vi "TEST_L1_INITIALISATION_CHECK.vi"(5 "Serial Number":string="testFile", 6 "error in":errorcluster, 9 "VISA IN":T1={"AWG VISA"="AgilentGenerator1", "Oscilloscope  VISA "="AgilentOsciloscope", "Integration Board IP"="172.16.17.48", "connection ID"=refnum, "report out"=refnum, "report file path"=path "C:/Users/omartinez/Desktop/L0nL1_Results"}) -> (0 "error out":errorcluster, 3 "VISA OUT":T1={"AWG VISA"="AgilentGenerator1", "Oscilloscope  VISA "="AgilentOsciloscope", "Integration Board IP"="172.16.17.48", "connection ID"=refnum, "report out"=refnum, "report file path"=path "C:/Users/omartinez/Desktop/L0nL1_Results"})   [LabVIEW 2012]
uses:
  <vilib>/Utility/NIReport.llb/NI_report.lvclass
  <vilib>/Utility/NIReport.llb/HTML/NI_HTML.lvclass
panel:
  in  "Default register":u16[](array[numeric])=[6826, 18761, 18761, 18761, 30576, 383, 13312]
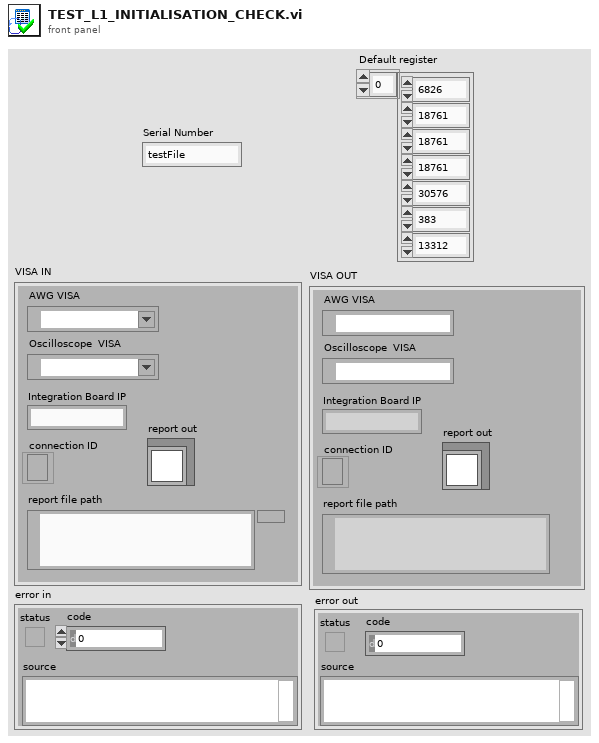
[diagram p1: front panel]
types:
  T1 = cluster{"AWG VISA":refnum<visa-resource-name>, "Oscilloscope  VISA ":refnum<visa-resource-name>, "Integration Board IP":string, "connection ID":refnum<k5>, "report out":refnum<class "NI_report.lvclass">, "report file path":path}
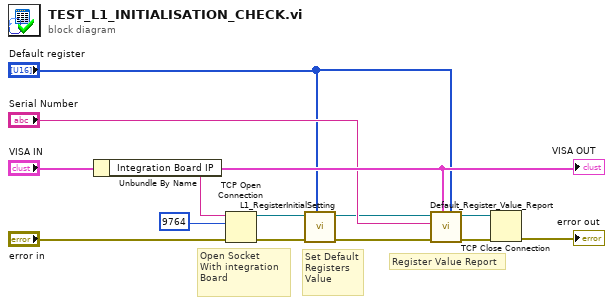
[diagram p0: block diagram]
diagram:
  # "Set Default\nRegisters\nValue"
  # "Open Socket\nWith integration \nBoard"
  # "Register Value Report"
  n1 = Unbundle By Name("VISA IN") -> ("Integration Board IP"=w8:string)
  n2 = TCP Open Connection(address=w8, remote port or service name=9764, error in (no error)="error in") -> (connection ID=w3:refnum<k5>, error out=w5:errorcluster)  [unwired: 2 in]
  n3 = call "L1_RegisterInitialSetting.vi"("REG ARRAy"="Default register", "error in"=w5, "connection ID in"=w3) -> ("error out"=w4:errorcluster, "connection ID out"=w2:refnum<k5>)  [unwired: 7 in]
  n4 = call "Default_Register_Value_Report.vi"("Default register"="Default register", "input cluster"="VISA IN", "error out"=w4, "Serial Number"="Serial Number", "connection ID"=w2) -> ("error out 2"=w11:errorcluster, "connection ID out"=w10:refnum<k5>)  [unwired: 4 in, 1 out]
  n5 = TCP Close Connection(connection ID=w10, error in (no error)=w11) -> (error out=→"error out":errorcluster)  [unwired: 1 in, 1 out]
  "VISA OUT" <- "VISA IN"
